vi "get_fav_cartoon.vi"() -> (4 "Cartoon out":T2, 6 "Back out":T1, 8 "path":path)   [LabVIEW 2023]
doc: "Get the cartoon character"
uses:
  custom_elements/fav_cartoon.ctl
  custom_elements/back_button.ctl
panel:
  in  "Back":T1
  in  "Shin_chan":bool caption="Shin Chan"
  in  "Tom_and_jerry":bool caption="Tom and jerry"
  in  "Ben_10":bool caption="Ben !0"
  in  "Pokemon":bool
  # "Select you favourite Cartoon"
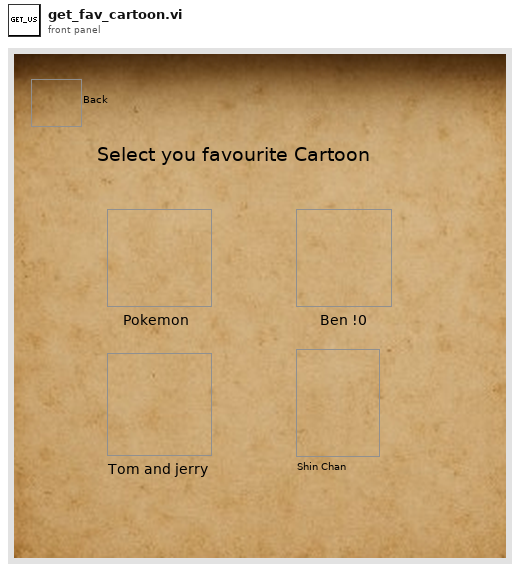
[diagram p1: front panel]
types:
  T1 = typedef "back_button.ctl" = bool
  T2 = typedef "fav_cartoon.ctl" = enum16{"Ben 10", "Shin Chan", "Pokemon", "Tom and Jerry"}
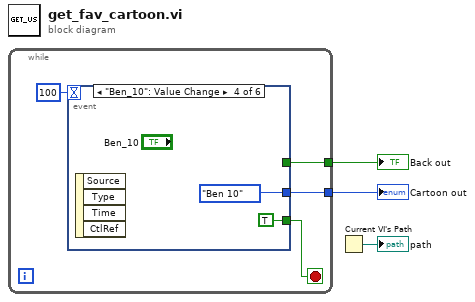
[diagram p0: block diagram]
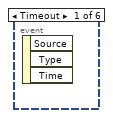
[diagram p2: hidden frame]
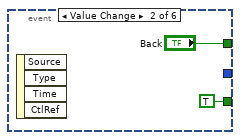
[diagram p3: hidden frame]
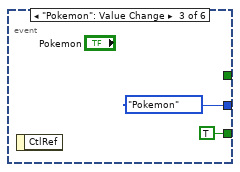
[diagram p4: hidden frame]
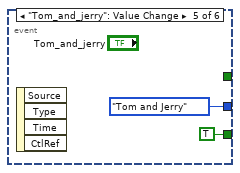
[diagram p5: hidden frame]
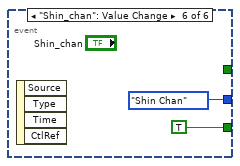
[diagram p6: hidden frame]
diagram:
  n1 = while {
    tunnel: [w5] -> w2
    tunnel: [w4] -> w1
    stop <- w6 stop-if-true
    n2 = event shown="[3] \"Ben_10\": Value Change" {
      selector: _ -> [_ _ _ _ _ _]
      dyn-events: _ -> [_ _ _ _ _ _]
      timeout: 100 -> [_ _ _ _ _ _]
      tunnel: [_ TRUE TRUE TRUE TRUE TRUE] -> w6
      tunnel: [_ _ fav_cartoon."Pokemon" fav_cartoon."Ben 10" fav_cartoon."Tom and Jerry" fav_cartoon."Shin Chan"] -> w5
      tunnel: [_ "Back" _ _ _ _] -> w4
      event Timeout {
        n3 = event-data() -> ()  [unwired: 1 in, 3 out]
      }
      event Value Change {
        n4 = event-data() -> ()  [unwired: 1 in, 4 out]
      }
      event "Pokemon": Value Change {
        n5 = event-data() -> ()  [unwired: 1 in, 1 out]
      }
      event "Ben_10": Value Change {
        n6 = event-data() -> ()  [unwired: 1 in, 4 out]
      }
      event "Tom_and_jerry": Value Change {
        n7 = event-data() -> ()  [unwired: 1 in, 4 out]
      }
      event "Shin_chan": Value Change {
        n8 = event-data() -> ()  [unwired: 1 in, 4 out]
      }
    }
  }
  "Cartoon out" <- w2
  "Back out" <- w1
  n9 = Current VI's Path() -> (path=→"path":path)
